vi "SysDef.Globals.vi"() -> ()   [LabVIEW 2015, in "Import - Export CD Config Utility.lvlib"]
uses:
  Import - Export CD Config Utility.lvlib
panel:
  in  "Version":string="1.0.0"
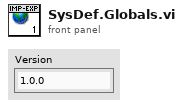
[diagram p1: front panel]
diagram:
